vi "GT Get Clock.vi"(8 "error in (no error)":errorcluster caption="错误输入（无错误）", 9 "pLoop":u32, 10 "pClock":u32, 11 "cardNum":i16) -> (0 "error out":errorcluster caption="错误输出", 1 "pLoop out":u32, 2 "pClock out":u32, 3 "function return":i16)   [LabVIEW 2014, in "gts.lvlib"]
doc: "GT_API GT_GetClock(short cardNum,unsigned long *pClock,unsigned long *pLoop=NULL);"
uses:
  gts.lvlib
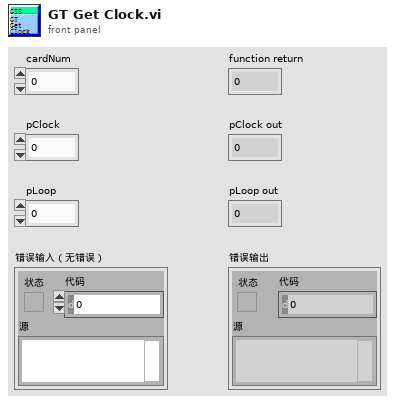
[diagram p1: front panel]
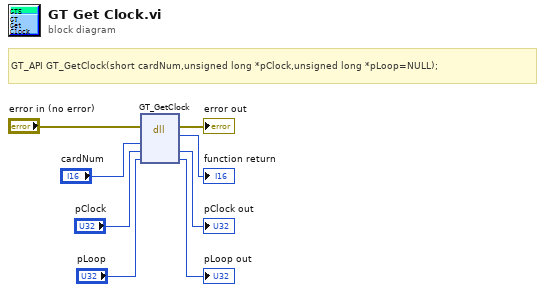
[diagram p0: block diagram]
diagram:
  # "GT_API GT_GetClock(short cardNum,unsigned long *pClock,unsigned long *pLoop=NULL);"
  n1 = dll-call lib="PTH2habs D固高科技资料GTS控制卡GTS卡18年上半年资料dllVC32bit\nmulti_cardgts.*" fn="GT_GetClock"(error in="error in (no error)", "cardNum"="cardNum", "pClock"="pClock", "pLoop"="pLoop") -> (error out=→"error out":errorcluster, →"function return":i16, "pClock"=→"pClock out":u32, "pLoop"=→"pLoop out":u32)  [unwired: 3 in, 1 out]
